vi "TSLIN_Process_Asyn_Call.vi"(8 "错误输入":errorcluster, 9 "Queue Name":string, 10 "Ref_Arry":refnum<vi>[](array[refnum]), 11 "Data":T1={"Communication message"={"Sender"="", "receiver"="", "message"="", "data"=variant}, "LIN_Data"={"DLL_PATH"=path "", "Channels used"=1, "Funtiontype"=0, "Rx/TX"=enum."Rx", "Read message type"=enum."Receive&send messages", "async&sync"=enum."async", "sync_sendTimeout"=0, "LIN_SendHead"={"ALINIdxchn"=0, "ALINId"=0, "ALINDLC"=0}, "LIN_Set"={"Hardware Type"=2, "Hardware Subtype"=enum."TC1016", "AHwChannel"=0, "AAppChannel"=19, "ABaudrateKbps"=19.2, "AProtocol"=2, "AldHW"=0}, "LIN_DATA"={"Data0"=0, "Data1"=0, "Data2"=0, "Data3"=0, "Data4"=0, "Data5"=0, "Data6"=0, "Data7"=0}, "LIN_Set_Array"=[], "LDF"={"LDF Path"=path "", "LDF loading channel"=0}, "Blf_Log"={"Blf_Log_PATH"=path ""}, "LIN Scheduling Table Array"=[], "REC_Channel"=0}, "LIN Data array"=[], "error in"={"status"=FALSE, "code"=0, "source"=""}, "REC_Channel"=0, "AsynCall?"=FALSE, "DataBase_array"=refnum} {"REC_Channel" items=["CHN1", "CHN2", "CHN3", "CHN4", "CHN5", "CHN6", "CHN7", "CHN8", "CHN9", "CHN10", "CHN11", "CHN12", "CHN13", "CHN14", "CHN15", "CHN16", "CHN17", "CHN18", "CHN19", "CHN20", "CHN21", "CHN22", "CHN23", "CHN24", "CHN25", "CHN26", "CHN27", "CHN28", "CHN29", "CHN30", "CHN31", "CHN32"]; "LIN_Data"."REC_Channel" items=["CHN1", "CHN2", "CHN3", "CHN4", "CHN5", "CHN6", "CHN7", "CHN8", "CHN9", "CHN10", "CHN11", "CHN12", "CHN13", "CHN14", "CHN15", "CHN16", "CHN17", "CHN18", "CHN19", "CHN20", "CHN21", "CHN22", "CHN23", "CHN24", "CHN25", "CHN26", "CHN27", "CHN28", "CHN29", "CHN30", "CHN31", "CHN32"]; "LIN_Data"."LIN Scheduling Table Array"."LIN_Transmit"."Channel" items=["CHN1", "CHN2", "CHN3", "CHN4", "CHN5", "CHN6", "CHN7", "CHN8", "CHN9", "CHN10", "CHN11", "CHN12", "CHN13", "CHN14", "CHN15", "CHN16", "CHN17", "CHN18", "CHN19", "CHN20", "CHN21", "CHN22", "CHN23", "CHN24", "CHN25", "CHN26", "CHN27", "CHN28", "CHN29", "CHN30", "CHN31", "CHN32"]; "LIN_Data"."LIN Scheduling Table Array"."LIN_Transmit"."ID" format="%.0x"; "LIN_Data"."LIN Scheduling Table Array"."LIN_Transmit"."DLC" format="%.0x"; "LIN_Data"."LIN Scheduling Table Array"."LIN_Transmit"."Set_node_funtiontype" items=["MasterNode", "SlaveNode", "MonitorNote"]; "LIN_Data"."LDF"."LDF loading channel" items=["CHN1", "CHN2", "CHN3", "CHN4", "CHN5", "CHN6", "CHN7", "CHN8", "CHN9", "CHN10", "CHN11", "CHN12", "CHN13", "CHN14", "CHN15", "CHN16", "CHN17", "CHN18", "CHN19", "CHN20", "CHN21", "CHN22", "CHN23", "CHN24", "CHN25", "CHN26", "CHN27", "CHN28", "CHN29", "CHN30", "CHN31", "CHN32"]; "LIN_Data"."LIN_Set_Array"."Set_node_funtiontype" items=["MasterNode", "SlaveNode", "MonitorNote"]; "LIN_Data"."LIN_Set_Array"."Set"."Hardware Type" items=["BUS_UNKNOWN_TYPE", "TS_TCP_DEVICE", "XL_USB_DEVICE", "TS_USB_DEVICE", "PEAK_USB_DEVICE", "KVASER_USB_DEVICE", "ZLG_USB_DEVICE", "ICS_USB_DEVICE", "TS_TC1005_DEVICE", "CANABLE_USB_DEVICE", "TS_WIRELESS_OBD", "TS_USB_DEVICE_EX", "IXXAT_USB_DEVICE", "TS_ETH_IF_DEVICE", "TS_USB_IF_DEVICE", "BUS_DEV_TYPE_COUNT"]; "LIN_Data"."LIN_Set_Array"."Set"."AHwChannel" items=["CHN1", "CHN2", "CHN3", "CHN4", "CHN5", "CHN6", "CHN7", "CHN8", "CHN9", "CHN10", "CHN11", "CHN12", "CHN13", "CHN14", "CHN15", "CHN16", "CHN17", "CHN18", "CHN19", "CHN20", "CHN21", "CHN22", "CHN23", "CHN24", "CHN25", "CHN26", "CHN27", "CHN28", "CHN29", "CHN30", "CHN31", "CHN32"]; "LIN_Data"."LIN_Set_Array"."Set"."AAppChannel" items=["CHN1", "CHN2", "CHN3", "CHN4", "CHN5", "CHN6", "CHN7", "CHN8", "CHN9", "CHN10", "CHN11", "CHN12", "CHN13", "CHN14", "CHN15", "CHN16", "CHN17", "CHN18", "CHN19", "CHN20", "CHN21", "CHN22", "CHN23", "CHN24", "CHN25", "CHN26", "CHN27", "CHN28", "CHN29", "CHN30", "CHN31", "CHN32"]; "LIN_Data"."LIN_Set_Array"."Set"."AProtocol" items=["Lin_Protocol_13", "Lin_Protocol_20", "Lin_Protocol_21", "Lin_Protocol_J2602"]; "LIN_Data"."Funtiontype" items=["MasterNode", "SlaveNode", "MonitorNote"]; "LIN_Data"."LIN_SendHead"."ALINDLC" format="%.0x"; "LIN_Data"."LIN_SendHead"."ALINId" format="%.0x"; "LIN_Data"."LIN_SendHead"."ALINIdxchn" items=["CHN1", "CHN2", "CHN3", "CHN4", "CHN5", "CHN6", "CHN7", "CHN8", "CHN9", "CHN10", "CHN11", "CHN12", "CHN13", "CHN14", "CHN15", "CHN16", "CHN17", "CHN18", "CHN19", "CHN20", "CHN21", "CHN22", "CHN23", "CHN24", "CHN25", "CHN26", "CHN27", "CHN28", "CHN29", "CHN30", "CHN31", "CHN32"]; "LIN_Data"."LIN_Set"."Hardware Type" items=["BUS_UNKNOWN_TYPE", "TS_TCP_DEVICE", "XL_USB_DEVICE", "TS_USB_DEVICE", "PEAK_USB_DEVICE", "KVASER_USB_DEVICE", "ZLG_USB_DEVICE", "ICS_USB_DEVICE", "TS_TC1005_DEVICE", "CANABLE_USB_DEVICE", "TS_WIRELESS_OBD", "TS_USB_DEVICE_EX", "IXXAT_USB_DEVICE", "TS_ETH_IF_DEVICE", "TS_USB_IF_DEVICE", "BUS_DEV_TYPE_COUNT"]; "LIN_Data"."LIN_Set"."AHwChannel" items=["CHN1", "CHN2", "CHN3", "CHN4", "CHN5", "CHN6", "CHN7", "CHN8", "CHN9", "CHN10", "CHN11", "CHN12", "CHN13", "CHN14", "CHN15", "CHN16", "CHN17", "CHN18", "CHN19", "CHN20", "CHN21", "CHN22", "CHN23", "CHN24", "CHN25", "CHN26", "CHN27", "CHN28", "CHN29", "CHN30", "CHN31", "CHN32"]; "LIN_Data"."LIN_Set"."AAppChannel" items=["CHN1", "CHN2", "CHN3", "CHN4", "CHN5", "CHN6", "CHN7", "CHN8", "CHN9", "CHN10", "CHN11", "CHN12", "CHN13", "CHN14", "CHN15", "CHN16", "CHN17", "CHN18", "CHN19", "CHN20", "CHN21", "CHN22", "CHN23", "CHN24", "CHN25", "CHN26", "CHN27", "CHN28", "CHN29", "CHN30", "CHN31", "CHN32"]; "LIN_Data"."LIN_Set"."AProtocol" items=["Lin_Protocol_13", "Lin_Protocol_20", "Lin_Protocol_21", "Lin_Protocol_J2602"]; "LIN_Data"."Channels used" items=["1 Channel"=1, "2 Channels"=2, "3 Channels"=3, "4 Channels"=4, "5 Channels"=5]}) -> (0 "error out":errorcluster)   [LabVIEW 2014]
uses:
  Utilities/Typedef/Hardware_Subtype.ctl
  Typedef/TSLIN_SetData.ctl
  Typedef/TSLIN_SendHead.ctl
  Typedef/TSLIN_Config.ctl
  Typedef/TLibLIN.ctl
  Typedef/TSLIN_Data.ctl
  Typedef/TSLIN_Transmit.ctl
  Typedef/TSLIN_LIN Schedule_Table.ctl
  Typedef/TSLIN_LIN_Set.ctl
  All_Control/Typedef/Hardware Type.ctl
  All_Control/Typedef/Blf_Log.ctl
  DataBase/Typedef/CAN/TCANSignal.ctl
  DataBase/Typedef/LIN/TLINSignal.ctl
  DataBase/Typedef/FlexRay/TFlexRaySignal.ctl
  DataBase/Typedef/TDBSignalProperties.ctl
  DataBase/Typedef/TDBFrameProperties.ctl
  DataBase/Typedef/TDBECUProperties.ctl
  DataBase/Typedef/TDBProperties.ctl
  DataBase/Typedef/DataBase_array.ctl
  DataBase/Typedef/DataBase_array_index.ctl
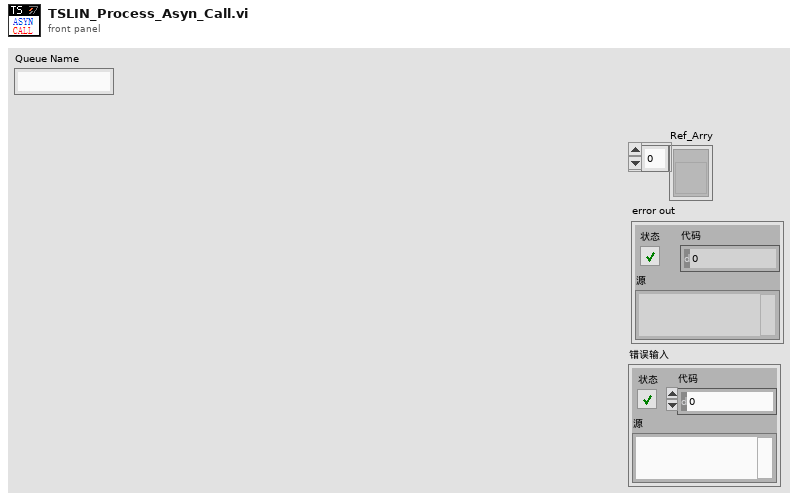
[diagram p1: front panel]
types:
  T1 = typedef "TSLIN_Data.ctl" = cluster{"Communication message":cluster{"Sender":string, "receiver":string, "message":string, "data":variant}, "LIN_Data":T2, "LIN Data array":T11[], "error in":errorcluster, "REC_Channel":i32, "AsynCall?":bool, "DataBase_array":T12}
  T2 = typedef "TSLIN_Config.ctl" = cluster{"DLL_PATH":path, "Channels used":u16, "Funtiontype":i32, "Rx/TX":enum16{"Rx", "Tx"}, "Read message type":enum16{"Only read received messages", "Receive&send messages"}, "async&sync":enum16{"async", "sync"}, "sync_sendTimeout":u16, "LIN_SendHead":T3, "LIN_Set":T4, "LIN_DATA":cluster{"Data0":u8, "Data1":u8, "Data2":u8, "Data3":u8, "Data4":u8, "Data5":u8, "Data6":u8, "Data7":u8}, "LIN_Set_Array":T7[], "LDF":cluster{"LDF Path":path, "LDF loading channel":i32}, "Blf_Log":T8, "LIN Scheduling Table Array":T9[], "REC_Channel":i32}
  T3 = typedef "TSLIN_SendHead.ctl" = cluster{"ALINIdxchn":u8, "ALINId":u32, "ALINDLC":u32}
  T4 = typedef "TSLIN_SetData.ctl" = cluster{"Hardware Type":T5, "Hardware Subtype":T6, "AHwChannel":i32, "AAppChannel":i32, "ABaudrateKbps":sgl, "AProtocol":i32, "AldHW":i32}
  T5 = typedef "Hardware Type.ctl" = i32
  T6 = typedef "Hardware_Subtype.ctl" = enum16{"TS_UNKNOWN_DEVICE", "TSCAN_PRO", "TSCAN_Lite1", "TC1001", "TL1001", "TC1011", "TM5011", "TC1002", "TC1014", "TSCANFD2517", "TC1026", "TC1016", "TC1012", "TC1013", "TLog1002", "TC1034", "TC1018", "GW2116", "TC2115", "MP1013", "TC1113", "TC1114", "TP1013", "TC1017", "TP1018", "TF10XX", "TL1004_FD_4_LIN_2", "TE1051", "TP1051", "TP1034", "TTS9015", "TP1026", "TTS1026", "TTS1034", "TTS1018", "TL1011", "TTS1015_LiAuto", "TTS1013_LiAuto", "TTS1016Pro", "TC1054Pro", "TC1054", "TLog1038", "TO1013", "TC1034Pro", "TC1018Pro", "TC1038Pro", "TS_DEV_END"}
  T7 = typedef "TSLIN_LIN_Set.ctl" = cluster{"Set":T4, "Set_node_funtiontype":i32}
  T8 = typedef "Blf_Log.ctl" = cluster{"Blf_Log_PATH":path}
  T9 = typedef "TSLIN_LIN Schedule_Table.ctl" = cluster{"LIN_Transmit":T10, "Delay(ms)":i32}
  T10 = typedef "TSLIN_Transmit.ctl" = cluster{"Channel":i32, "Rx/TX":enum16{"Rx", "Tx"}, "Set_node_funtiontype":i32, "DLC":u32, "ID":u32, "FDatas":cluster{"value0":u8, "value 1":u8, "value 2":u8, "value 3":u8, "value 4":u8, "value 5":u8, "value 6":u8, "value 7":u8}}
  T11 = typedef "TLibLIN.ctl" = cluster{"Ch":u8, "Code":u8, "Properties":u8, "FDLC":u8, "ID":u8, "Checksum":u8, "FStaus":u8, "FTimeUS":u64, "FDatas":cluster{"value0":u8, "value 1":u8, "value 2":u8, "value 3":u8, "value 4":u8, "value 5":u8, "value 6":u8, "value 7":u8}}
  T12 = typedef "DataBase_array_index.ctl" = refnum<vi>
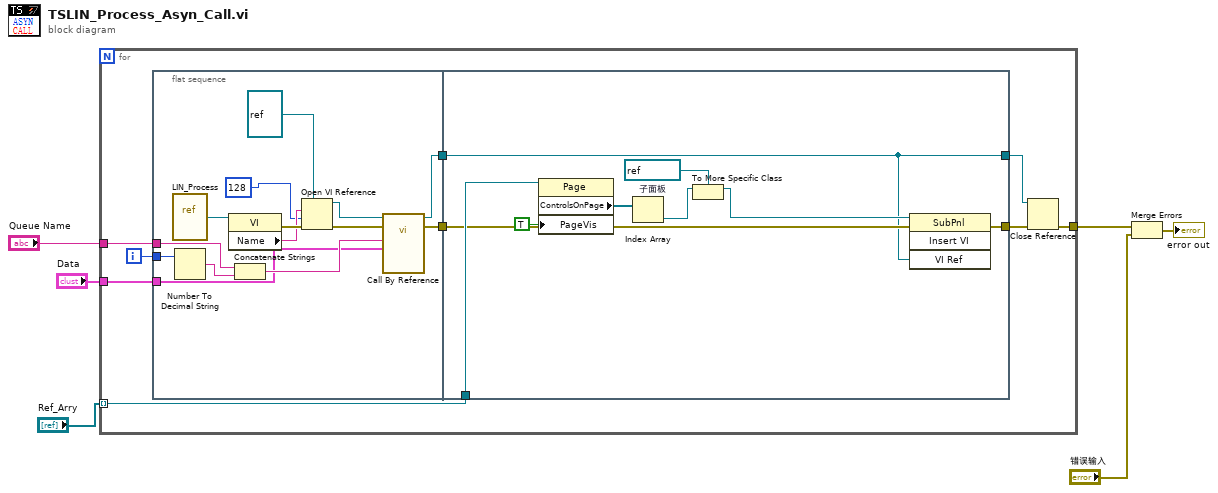
[diagram p0: block diagram]
diagram:
  n1 = for {
    tunnel: "Queue Name" -> [w12]
    tunnel: "Data" -> [w11]
    tunnel: "Ref_Arry" -> [w8] mode=indexing
    tunnel: [w7] -> w3
    i -> [w13]
    n2 = flat-sequence {
      tunnel: w13 -> [w21]
      tunnel: w12 -> [w19]
      tunnel: w11 -> [w16]
      tunnel: [w27] -> w10
      tunnel: [w26] -> w9
      tunnel: [w32] -> w14
      tunnel: [w31] -> w15
      tunnel: w10 -> [w31]
      tunnel: w9 -> [w33]
      tunnel: w8 -> [w35]
      frame #0 {
        n3 = vi-ref "LIN_Process.vi"() -> (w22:refnum<vi>)
        n4 = Number To Decimal String(number=w21) -> (decimal integer string=w20:string)  [unwired: 1 in]
        n5 = property class="VI"(reference=w22) -> (error out=w29:errorcluster, "Name"=w23:string)  [unwired: 1 in, 1 out]
        n6 = Concatenate Strings(w19, w20) -> (w18:string)
        n7 = Open VI Reference(type specifier VI Refnum (for type only)=refnum<vi> refnum ("类型说明符VI引用句柄（仅用于类型）"), vi path=w23, options=128 ("选项"), error in (no error)=w29) -> (vi reference=w25:refnum<vi>, error out=w28:errorcluster)  [unwired: 2 in]
        n8 = call-by-ref "?"(reference=w25, error in=w28, "Data"=w16, "Queue Name"=w18) -> (reference out=w27:refnum<vi>, error out=w26:errorcluster)  [unwired: 10 in]
      }
      frame #1 {
        w36 = refnum<vi> refnum  # 子面板
        n9 = property class="Page"(reference=w35, "PageVis"=TRUE ("选项卡可见")) -> ("ControlsOnPage"=w38:refnum<vi>[])  [unwired: 1 in, 2 out]
        n10 = Index Array(array=w38) -> (element=w37:refnum<vi>)  [unwired: 1 in]
        n11 = To More Specific Class(target class=w36, reference=w37) -> (specific class reference=w34:refnum<vi>)  [unwired: 1 in, 1 out]
        n12 = invoke class="SubPnl" method="Insert VI"(reference=w34, error in=w33, "VI Ref"=w31) -> (error out=w32:errorcluster)  [unwired: 1 in, 3 out]
      }
    }
    n13 = Close Reference(reference=w15, error in (no error)=w14) -> (error out=w7:errorcluster)
  }
  n14 = Merge Errors(w3, "错误输入") -> (→"error out":errorcluster)
